vi "温度曲线写入.vi"(8 "error in (no error)":errorcluster caption="错误输入（无错误）", 10 "data":T1={"时间"=timestamp(0 s since 1904-01-01), "测量模式"="水样测试", "数据类型"="N", "检测值"=0.0, "单位"="mg/L", "数据标识"="N", "X"=0.0, "量程标识"="", "SN"="", "标样参考值"=0.0, "跨度值"=0.0, "F0"=0.0, "F1"=0.0, "F2"=0.0, "F3"=0.0, "F4"=0.0, "F5"=0.0, "F6"=0.0, "F7"=0.0, "X1"=0.0, "因子编码"="", "温度"=0.0, "湿度"=0.0, "测量量程"=0.0, "测量检出限"=0.0, "测量精度"=0.0, "测量间隔"=0.0, "消解温度"=0.0, "消解时长"=0.0, "三项式系数"=0.0, "二次多项式系数"=0.0, "曲线斜率"=0.0, "曲线截距"=0.0, "线性相关系数"=0.0, "空白校准时间"=timestamp(0 s since 1904-01-01), "标样校准时间"=timestamp(0 s since 1904-01-01), "测量信号值"=0.0, "稀释倍数"=0.0, "空白标定系数"=0.0, "量程系数"=0.0, "LastTime"=timestamp(0 s since 1904-01-01)}, 11 "table":string="总氮") -> (0 "错误输出":errorcluster)   [LabVIEW 2016, in "斯坦道总磷总氮V2.lvlib"]
uses:
  <vilib>/Utility/VariantDataType/VariantType.lvlib
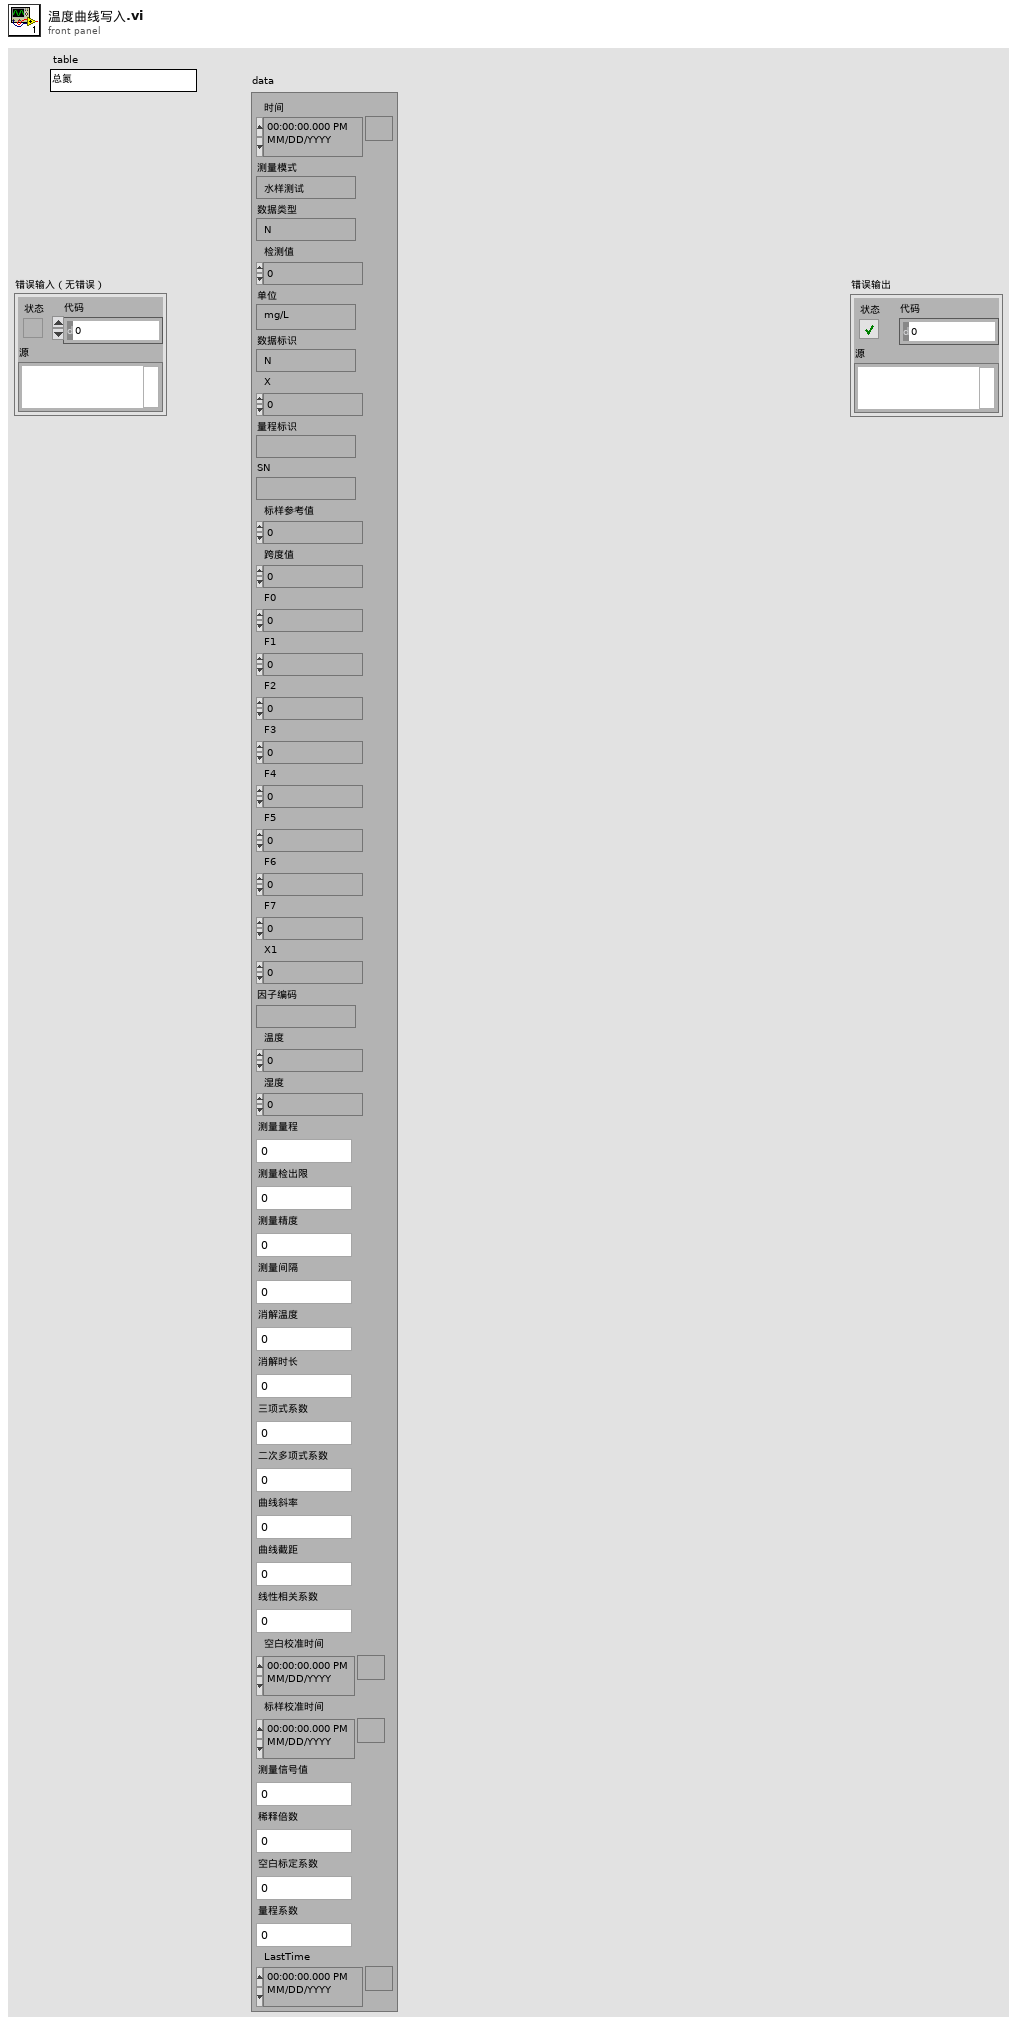
[diagram p1: front panel]
types:
  T1 = typedef "营养盐字段定义.ctl" = cluster{"时间":timestamp, "测量模式":string, "数据类型":string, "检测值":sgl, "单位":string, "数据标识":string, "X":sgl, "量程标识":string, "SN":string, "标样参考值":sgl, "跨度值":sgl, "F0":sgl, "F1":sgl, "F2":sgl, "F3":sgl, "F4":sgl, "F5":sgl, "F6":sgl, "F7":sgl, "X1":sgl, "因子编码":string, "温度":sgl, "湿度":sgl, "测量量程":sgl, "测量检出限":sgl, "测量精度":sgl, "测量间隔":sgl, "消解温度":sgl, "消解时长":sgl, "三项式系数":sgl, "二次多项式系数":sgl, "曲线斜率":sgl, "曲线截距":sgl, "线性相关系数":sgl, "空白校准时间":timestamp, "标样校准时间":timestamp, "测量信号值":sgl, "稀释倍数":sgl, "空白标定系数":sgl, "量程系数":sgl, "LastTime":timestamp}
  T2 = enum16{"open", "open or create", "create or replace", "create", "open (read-only)"}
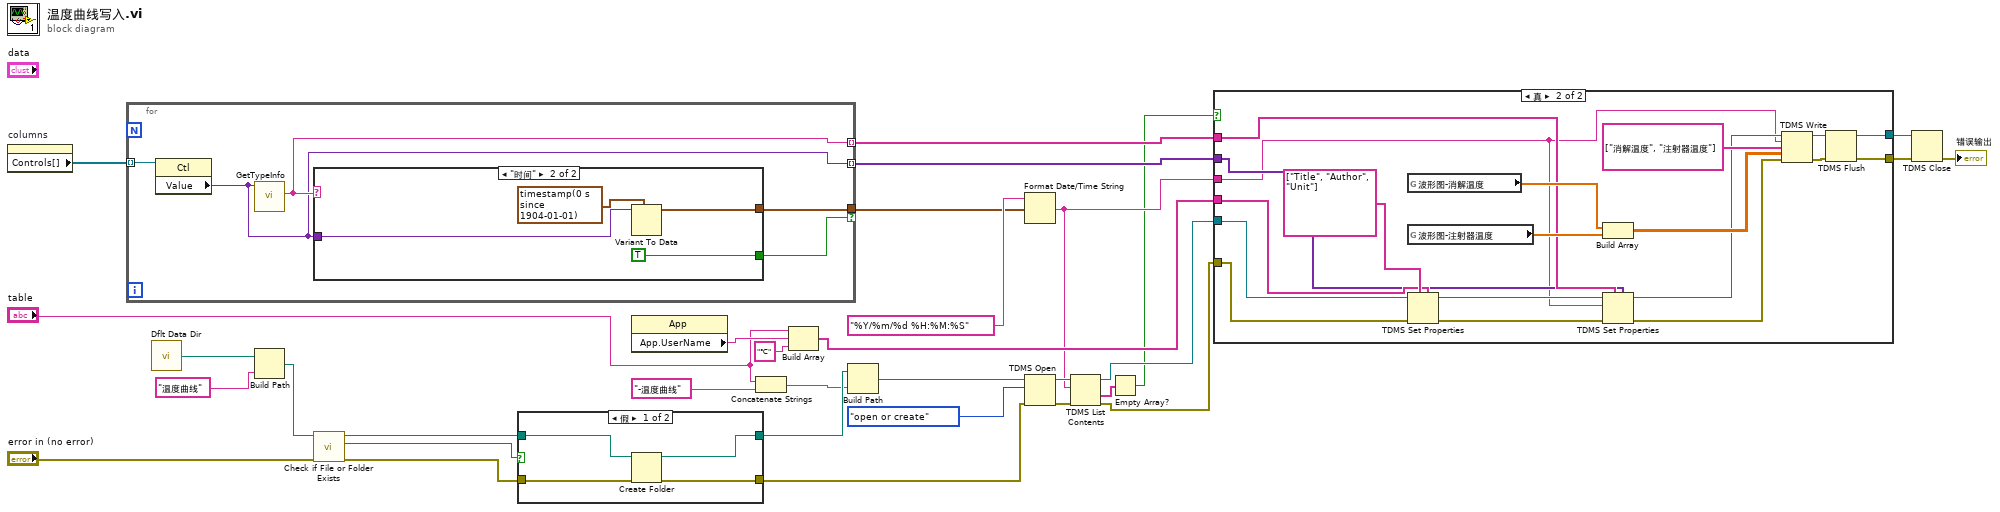
[diagram p0: block diagram]
diagram:
  n1 = property on="columns" class="Clust (严格)"() -> ("Controls[]"=w7:refnum<vi>[])  [unwired: 2 in, 2 out]
  n2 = for {
    tunnel: [w33] -> w9 mode=indexing
    tunnel: [w37] -> w10 mode=indexing
    tunnel: [w36] -> w8 if=w35
    tunnel: w7 -> [w34] mode=indexing
    n3 = property class="Ctl"(reference=w34) -> ("Value"=w33:variant)  [unwired: 1 in, 2 out]
    n4 = call <vilib>:"GetTypeInfo.vi"("Variant"=w33) -> ("Name"=w37:string)  [unwired: 6 in, 4 out]
    n5 = case shown="\"时间\"" w37 {
      tunnel: w33 -> [_ w41]
      tunnel: [_ w39] -> w36
      tunnel: [_ TRUE] -> w35
      frame "假", Default {
      }
      frame "时间" {
        n6 = Variant To Data(type=timestamp(0 s since 1904-01-01) ("时间标识"), Variant=w41) -> (data=w39:timestamp)  [unwired: 1 in, 1 out]
      }
    }
  }
  n7 = call <vilib>:"Dflt Data Dir.vi"() -> ("App:Default Data Directory"=w27:path)
  n8 = Build Path(base path=w27, name or relative path="温度曲线" ("名称或相对路径")) -> (appended path=w25:path)
  n9 = call <vilib>:"Check if File or Folder Exists.vi"("error in (no error)"="error in (no error)", "path"=w25) -> ("error out"=w22:errorcluster, "file or folder exists?"=w24:bool, "dup path"=w23:path)  [unwired: 7 in]
  n10 = case shown="假" w24 {
    tunnel: w23 -> [w45 w46]
    tunnel: [w44 w46] -> w21
    tunnel: w22 -> [w43 w47]
    tunnel: [w42 w47] -> w15
    frame False {
      n11 = Create Folder(path (use dialog)=w45, error in=w43) -> (created path=w44:path, error out=w42:errorcluster)  [unwired: 1 in, 1 out]
    }
    frame True {
    }
  }
  n12 = property class="App"() -> ("App.UserName"=w31:string)  [unwired: 2 in, 2 out]
  n13 = Concatenate Strings("table", "-温度曲线" ("字符串")) -> (w19:string)
  n14 = Build Array("table", w31, "℃" ("元素")) -> (w30:string[])
  n15 = Build Path(base path=w21, name or relative path=w19) -> (appended path=w18:path)
  n16 = Format Date/Time String(time format string (%c)="%Y/%m/%d %H:%M:%S" ("时间格式字符串(%c)"), seconds (now)=w8) -> (date/time string=w3:string)  [unwired: 1 in]
  n17 = TDMS Open(8:w15, 10:T2."open or create" ("操作(0:open)"), 11:w18) -> (0:w32:errorcluster, 3:w5:refnum<k34>)  [unwired: 4 in]
  n18 = TDMS List Contents(4:w32, 6:w3, 7:w5) -> (0:w6:errorcluster, 1:w2:string[], 3:w4:refnum<k34>)  [unwired: 1 out]
  n19 = Empty Array?(array=w2) -> (empty?=w1:bool)
  n20 = case shown="真" w1 {
    tunnel: w30 -> [_ w67]
    tunnel: [w49 w57] -> w12
    tunnel: [w48 w56] -> w11
    tunnel: w10 -> [_ w54]
    tunnel: w9 -> [_ w53]
    tunnel: w6 -> [w49 w52]
    tunnel: w4 -> [w48 w51]
    tunnel: w3 -> [_ w50]
    frame False {
    }
    frame True {
      n21 = global read "VAR总磷总氮全局变量.vi" "波形图-消解温度"() -> (w64:dbl[])
      n22 = global read "VAR总磷总氮全局变量.vi" "波形图-注射器温度"() -> (w63:dbl[])
      n23 = TDMS Set Properties(5:w67, 7:string[] ["Title", "Author", "Unit"] ("property names"), 8:w52, 11:w51) -> (0:w62:errorcluster, 3:w55:refnum<k34>)  [unwired: 2 in, 2 out]
      n24 = Build Array(w64, w63) -> (w66:dbl[][])
      n25 = TDMS Set Properties(5:w53, 7:w54, 8:w62, 10:w50, 11:w55) -> (0:w61:errorcluster, 3:w60:refnum<k34>)  [unwired: 1 in, 2 out]
      n26 = TDMS Write(0:w60, 5:w50, 7:string[] ["消解温度", "注射器温度"] ("通道名输入（无标题）"), 9:w66, 11:w61) -> (4:w59:refnum<k34>, 15:w58:errorcluster)  [unwired: 1 in, 2 out]
      n27 = TDMS Flush(4:w58, 7:w59) -> (0:w57:errorcluster, 3:w56:refnum<k34>)
    }
  }
  n28 = TDMS Close(8:w12, 11:w11) -> (0:→"错误输出":errorcluster)  [unwired: 1 out]
